vi "InsituAcquire.vi"(8 "error in (no error)":errorcluster, 11 "Instruments in":refnum<class "Instruments.lvclass">) -> (0 "error out":errorcluster, 2 "output cluster":cluster{"Power":dbl, "Wl":dbl, "Voltage":dbl}, 3 "Instruments out":refnum<class "Instruments.lvclass">, 5 "remeasure?":bool)   [LabVIEW 2012, in "Instruments.lvclass"]
uses:
  Instruments.lvclass
  Controls/TestData.ctl
  Controls/Measurement.ctl
  Controls/SpectrometerOphirSelector.ctl
  Instruments.lvclass/Instruments.ctl
  <instrlib>/Keithley 24XX/Public/Data/Read (Multiple Points).vi
  <instrlib>/Keithley 24XX/Keithley 24XX.lvlib
  <vilib>/Analysis/NI_AALBase.lvlib
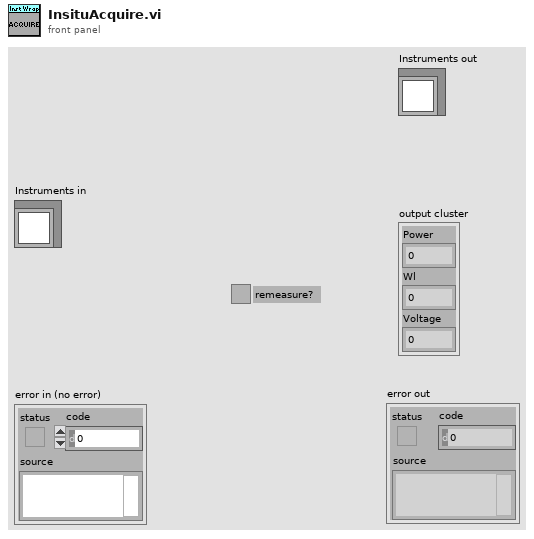
[diagram p1: front panel]
types:
  T1 = typedef "TestData.ctl" = cluster{"20mA Data":T2, "50mA Data ":T2}
  T2 = typedef "Measurement.ctl" = cluster{"Area":string, "Pad":string, "Current,mA":dbl, "Power":dbl, "WL":dbl, "Voltage":dbl, "Knee Current":dbl, "Reverse":dbl}
  T3 = typedef "SpectrometerOphirSelector.ctl" = enum16{"Get Background", "Measure", "Measure50", "Raw"}
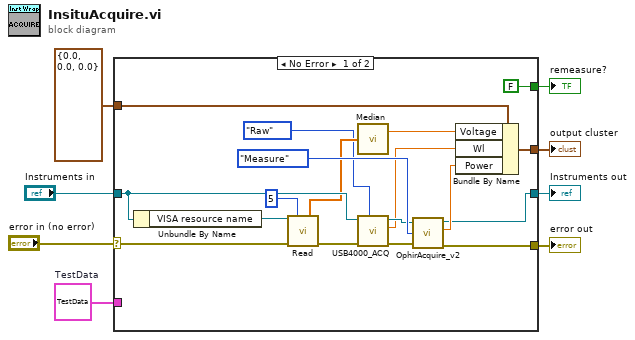
[diagram p0: block diagram]
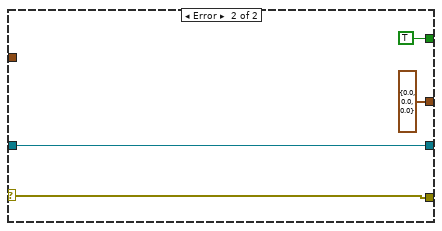
[diagram p2: hidden frame]
diagram:
  w5 = T1 {"20mA Data"={"Area"="", "Pad"="", "Current,mA"=0.0, "Power"=0.0, "WL"=0.0, "Voltage"=0.0, "Knee Current"=0.0, "Reverse"=0.0}, "50mA Data "={"Area"="", "Pad"="", "Current,mA"=0.0, "Power"=0.0, "WL"=0.0, "Voltage"=0.0, "Knee Current"=0.0, "Reverse"=0.0}}  # TestData
  n1 = case shown="No Error" "error in (no error)" {
    selector: "error in (no error)" -> [w25 w30]
    tunnel: [w12 w30] -> w8
    tunnel: [w11 w29] -> w6
    tunnel: "Instruments in" -> [w26 w29]
    tunnel: w5 -> [_ _]
    tunnel: [FALSE TRUE] -> w3
    tunnel: cluster{"Power":dbl, "Wl":dbl, "Voltage":dbl} {"Power"=0.0, "Wl"=0.0, "Voltage"=0.0} -> [w24 _]
    tunnel: [w14 cluster{"Power":dbl, "Wl":dbl, "Voltage":dbl} {"Power"=0.0, "Wl"=0.0, "Voltage"=0.0}] -> w1
    frame No Error {
      n2 = Unbundle By Name(w26) -> ("VISA resource name"=w21:refnum<visa-resource-name>)
      n3 = call-poly <instrlib>:"Read.vi"("VISA resource name"=w21, "Sample Count (1)"=5, "error in (no error)"=w25) -> ("Voltage"=w18:sgl[], "error out"=w19:errorcluster)  [unwired: 6 in, 5 out]
      n4 = call <vilib>:"Median.vi"("X"=w18) -> ("median"=w17:dbl)  [unwired: 1 out]
      n5 = call-dynamic "USB4000_ACQ.vi"("Type"=SpectrometerOphirSelector."Raw", "error in (no error)"=w19, "Instruments in"=w26) -> ("error out"=w20:errorcluster, "Peak Wl"=w16:dbl, "Instruments out"=w22:refnum<class "Instruments.lvclass">)  [unwired: 5 in, 1 out]
      n6 = call-dynamic "OphirAcquire_v2.vi"("Instruments in"=w22, "Type"=SpectrometerOphirSelector."Measure", "error in (no error)"=w20) -> ("Instruments out"=w11:refnum<class "Instruments.lvclass">, "Power,uW"=w15:dbl, "error out"=w12:errorcluster)  [unwired: 1 out]
      n7 = Bundle By Name(cluster=w24, "Voltage"=w17, "Wl"=w16, "Power"=w15) -> (w14:cluster{"Power":dbl, "Wl":dbl, "Voltage":dbl})
    }
    frame Error {
    }
  }
  "error out" <- w8
  "Instruments out" <- w6
  "remeasure?" <- w3
  "output cluster" <- w1
